vi "FTW-Reflection-Array.vi"(7 "Array":variant) -> (8 "Default Array Element":variant, 10 "Number of Dimensions":i32)   [LabVIEW 2012]
panel:
  # "Inputs"
  # "Outputs"
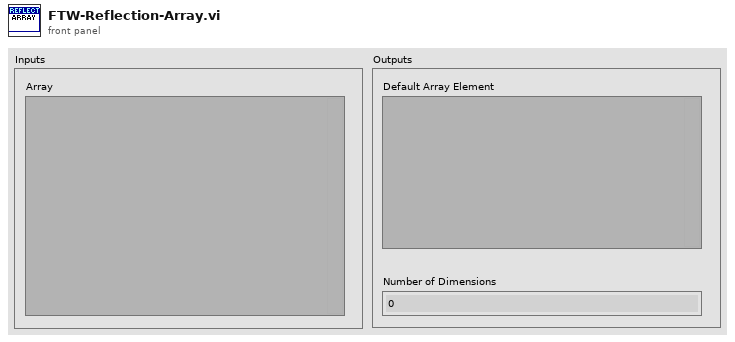
[diagram p1: front panel]
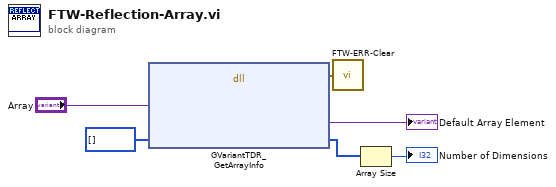
[diagram p0: block diagram]
diagram:
  n1 = dll-call lib="LabVIEW" fn="GVariantTDR_GetArrayInfo"("Array as a Variant"="Array", "Dimensions"=i32[] []) -> (error out=w4:errorcluster, "Default Array Element"=→"Default Array Element":variant, "Dimensions"=w2:i32[])  [unwired: 6 in, 1 out]
  n2 = call "FTW-ERR-Clear.vi"("error to snuff"=w4) -> ()  [unwired: 1 out]
  n3 = Array Size(array=w2) -> (size(s)=→"Number of Dimensions":i32)
